vi "IO_PumpCmdMsg18v7.vi"(6 "Enable":bool=TRUE, 8 "Drain Signal":bool, 9 "FIll Signal":bool, 10 "Pump Speed":enum16{"FAST", "SLOW", "CREEP", "STOP"}(ring)=enum."STOP", 11 "Cmd IN":u32=56) -> (0 "Pump State Out":enum16{"INIT", "IDLE", "STOP", "FILL", "DRAIN"}(ring)=enum."FILL", 1 "Msg Active":bool, 3 "Cmd Out":u32=80, 5 "ComCmd":string)   [LabVIEW 2024]
panel:
  # "D6(dir) D5(!en) D4(S1)  D3(S0) D2(X)  D1(X)  D0(X)   Dec\nSTOP   x       1        x      x       -     -      -        32\nINIT   1       1        1      1       -     -      -       120\nFILL   1       0        x      x       -     -      -        64\nDRAIN  0       0        x      x       -     -      -        00\n\nNONE   x       x        0      0       -     -      -        00    \nCREEP  x       x        0      1       -     -      -         8\nSLOW   x       x        1      0       -     -      -        16\nFAST   x       x        1      1       -     -      -        24"
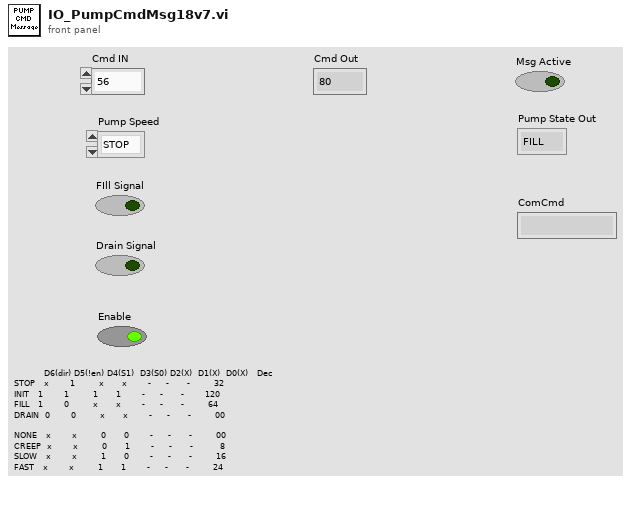
[diagram p1: front panel]
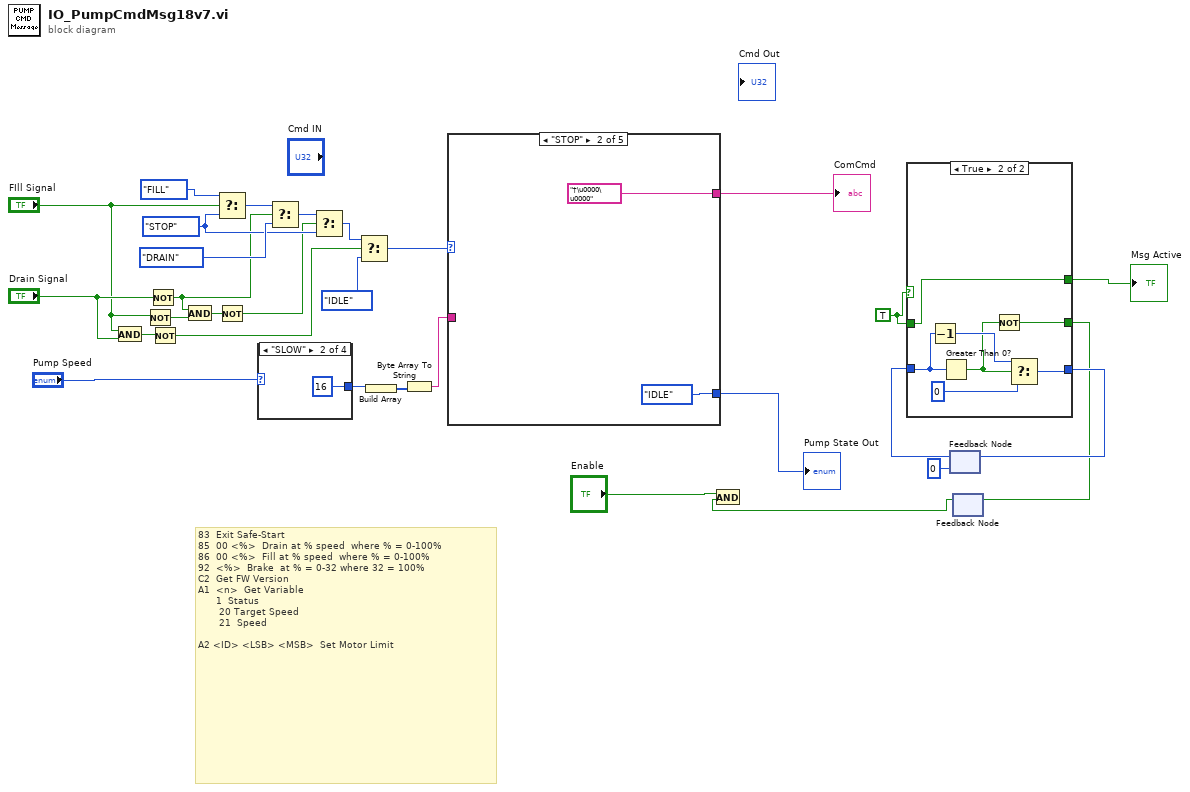
[diagram p0: block diagram]
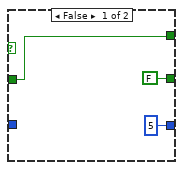
[diagram p2: hidden frame]
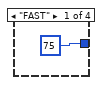
[diagram p3: hidden frame]
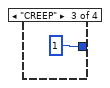
[diagram p4: hidden frame]
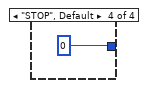
[diagram p5: hidden frame]
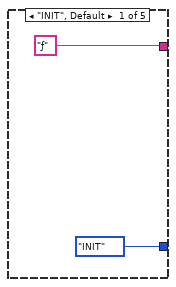
[diagram p6: hidden frame]
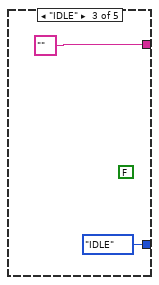
[diagram p7: hidden frame]
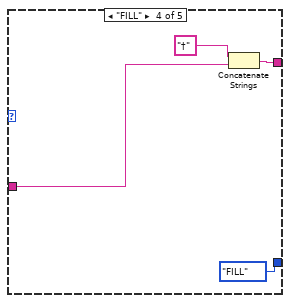
[diagram p8: hidden frame]
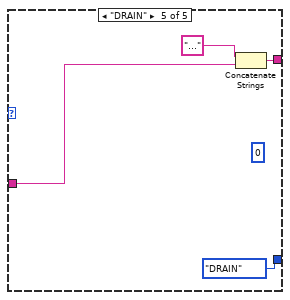
[diagram p9: hidden frame]
diagram:
  w1 = TRUE
  w26 = enum16{"INIT", "IDLE", "STOP", "FILL", "DRAIN"}."STOP" ("State")
  # "83  Exit Safe-Start\n85  00 <%>  Drain at % speed  where % = 0-100%\n86  00 <%>  Fill at % speed  where % = 0-100%\n92  <%>  Brake  at % = 0-32 where 32 = 100%\nC2  Get FW Version\nA1  <n>  Get Variable\n      1  Status\n       20 Target Speed\n       21  Speed\n\nA2 <ID> <LSB> <MSB>  Set Motor Limit"
  n1 = And(x="FIll Signal", y="Drain Signal") -> (x .and. y?=w14:bool)
  n2 = Not(x="FIll Signal") -> (.not. x?=w20:bool)
  n3 = Not(x="Drain Signal") -> (.not. x?=w19:bool)
  n4 = Not(x=w14) -> (.not. x?=w13:bool)
  n5 = And(x=w19, y=w20) -> (x .and. y?=w18:bool)
  n6 = Select(t=enum16{"INIT", "IDLE", "STOP", "FILL", "DRAIN"}."FILL" ("State"), s="FIll Signal", f=w26) -> (s? t:f=w29:enum16{"INIT", "IDLE", "STOP", "FILL", "DRAIN"})
  n7 = Not(x=w18) -> (.not. x?=w17:bool)
  n8 = case shown="\"SLOW\"" "Pump Speed" {
    tunnel: [u32 75 ("number") u32 16 ("number") u32 1 ("number") u32 0 ("number")] -> w4
    frame "FAST" {
    }
    frame "SLOW" {
    }
    frame "CREEP" {
    }
    frame "STOP", Default {
    }
  }
  n9 = Select(t=w29, s=w19, f=enum16{"INIT", "IDLE", "STOP", "FILL", "DRAIN"}."DRAIN" ("State")) -> (s? t:f=w27:enum16{"INIT", "IDLE", "STOP", "FILL", "DRAIN"})
  n10 = Select(t=w27, s=w17, f=w26) -> (s? t:f=w16:enum16{"INIT", "IDLE", "STOP", "FILL", "DRAIN"})
  n11 = Select(t=w16, s=w13, f=enum16{"INIT", "IDLE", "STOP", "FILL", "DRAIN"}."IDLE") -> (s? t:f=w12:enum16{"INIT", "IDLE", "STOP", "FILL", "DRAIN"})
  n12 = Build Array(w4) -> (w3:u32[])
  n13 = Byte Array To String(unsigned byte array=w3) -> (string=w2:string)
  n14 = case shown="\"STOP\"" w12 {
    tunnel: [enum16{"INIT", "IDLE", "STOP", "FILL", "DRAIN"}."INIT" ("State") enum16{"INIT", "IDLE", "STOP", "FILL", "DRAIN"}."IDLE" ("State") enum16{"INIT", "IDLE", "STOP", "FILL", "DRAIN"}."IDLE" ("State") enum16{"INIT", "IDLE", "STOP", "FILL", "DRAIN"}."FILL" ("State") enum16{"INIT", "IDLE", "STOP", "FILL", "DRAIN"}."DRAIN" ("State")] -> w22
    tunnel: ["ƒ" ("string") "†\u0000\u0000" "" w42 w46] -> w5
    tunnel: w2 -> [_ _ _ w41 w45]
    frame "INIT", Default {
    }
    frame "STOP" {
    }
    frame "IDLE" {
      (unwired) FALSE
    }
    frame "FILL" {
      n15 = Concatenate Strings("†" ("string"), w41) -> (w42:string)
    }
    frame "DRAIN" {
      (unwired) u32 0 ("number")
      n16 = Concatenate Strings("…" ("string"), w45) -> (w46:string)
    }
  }
  "Pump State Out" <- w22
  "ComCmd" <- w5
  n17 = feedback #1(0 ("f")) -> (w10:i32)
  n18 = case shown="True" w1 {
    tunnel: [w51 w52] -> w23
    tunnel: w1 -> [w51 w52]
    tunnel: [5 ("f") w55] -> w11
    tunnel: w10 -> [_ w53]
    tunnel: [FALSE w54] -> w8
    frame False {
    }
    frame True {
      n19 = Decrement(x=w53) -> (x-1=w58:i32)
      n20 = Greater Than 0?(x=w53) -> (x > 0?=w56:bool)
      n21 = Not(x=w56) -> (.not. x?=w54:bool)
      n22 = Select(t=w58, s=w56, f=0) -> (s? t:f=w55:i32)
    }
  }
  "Msg Active" <- w23
  n23 = feedback-in #1(w11) -> ()
  n24 = feedback-in #2(w8) -> ()
  n25 = feedback #2() -> (w7:bool)  [unwired: 1 in]
  n26 = And(x="Enable", y=w7) -> ()  [unwired: 1 out]
